vi "解码.vi"(1 "低8位":u8, 2 "中8位":u8, 3 "高8位":u8) -> (0 "输出":dbl)   [LabVIEW 2018]
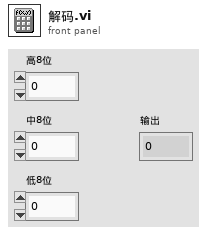
[diagram p1: front panel]
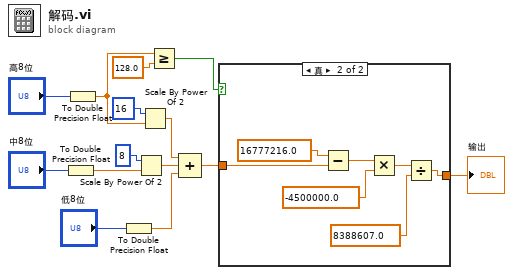
[diagram p0: block diagram]
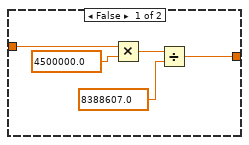
[diagram p2: hidden frame]
diagram:
  n1 = To Double Precision Float(number="中8位") -> (double precision float=w4:dbl)
  n2 = To Double Precision Float(number="高8位") -> (double precision float=w1:dbl)
  n3 = To Double Precision Float(number="低8位") -> (double precision float=w7:dbl)
  n4 = Scale By Power Of 2(n=i16 8, x=w4) -> (x*2^n=w12:dbl)
  n5 = Scale By Power Of 2(n=i16 16, x=w1) -> (x*2^n=w11:dbl)
  n6 = Greater Or Equal?(x=w1, y=128.0) -> (x >= y?=w9:bool)
  n7 = Compound Arithmetic op=ADD(w11, w12, w7) -> (w10:dbl)
  n8 = case shown="真" w9 {
    tunnel: w10 -> [w16 w25]
    tunnel: [w15 w20] -> w5
    frame False {
      n9 = Multiply(x=w16, y=4500000.0) -> (x*y=w18:dbl)
      n10 = Divide(x=w18, y=8388607.0) -> (x/y=w15:dbl)
    }
    frame True {
      n11 = Subtract(x=16777216.0, y=w25) -> (x-y=w24:dbl)
      n12 = Multiply(x=w24, y=-4500000.0) -> (x*y=w22:dbl)
      n13 = Divide(x=w22, y=8388607.0) -> (x/y=w20:dbl)
    }
  }
  "输出" <- w5
